vi "piezo2WriteOpen.vi"   [LabVIEW 2017]
uses:
  globalDevices.vi
  <vilib>/DAQmx/create/channels.llb/DAQmx Create Channel (AO-Voltage-Basic).vi
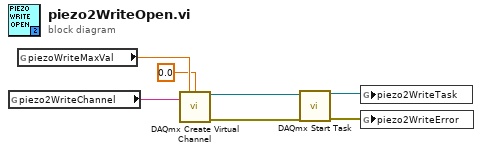
[diagram p0: block diagram]
diagram:
  n1 = global read "globalDevices.vi" "piezo2WriteChannel"() -> (w7:tag)
  n2 = global read "globalDevices.vi" "piezoWriteMaxVal"() -> (w6:dbl)
  n3 = call-poly <vilib>:"DAQmx Create Virtual Channel.vi"("maximum value"=w6, "minimum value"=0.0, "physical channels"=w7) -> ("task out"=w4:refnum<k21>, "error out"=w3:errorcluster)  [unwired: 11 in]
  n4 = call <vilib>:"DAQmx Start Task.vi"("task/channels in"=w4, "error in"=w3) -> ("task out"=w2:refnum<k21>, "error out"=w1:errorcluster)  [unwired: 12 in]
  n5 = global write "globalDevices.vi" "piezo2WriteTask"(w2) -> ()
  n6 = global write "globalDevices.vi" "piezo2WriteError"(w1) -> ()
